vi "n get waveform.vi"(7 "memptr":i16, 8 "error in (no error)":errorcluster, 9 "stopp":u16, 10 "channel":u16, 11 "n":u16) -> (0 "error out":errorcluster, 5 "memptr out":i16)   [LabVIEW 2015, in "SCANalone4x64.lvlib"]
doc: "__declspec(dllimport) void __stdcall n_get_waveform(unsigned short n, unsigned short channel, unsigned short stopp, signed short *memptr);"
uses:
  <userlib>/SCANalone4x64/SCANalone4x64.lvlib
  <userlib>/SCANalone4x64/SCANalone4x64.dll
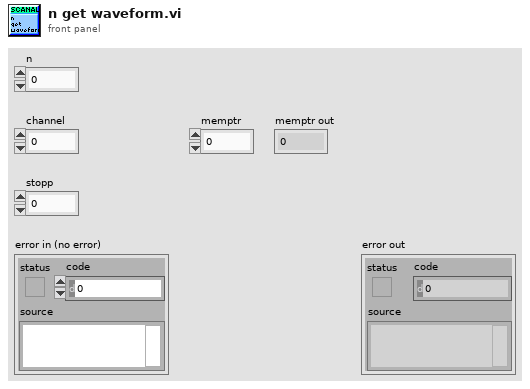
[diagram p1: front panel]
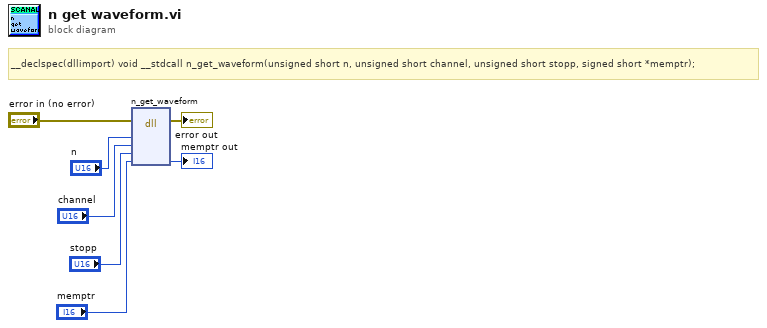
[diagram p0: block diagram]
diagram:
  # "__declspec(dllimport) void __stdcall n_get_waveform(unsigned short n, unsigned short channel, unsigned short stopp, signed short *memptr);"
  n1 = dll-call lib="C:/Program Files/National Instruments/LabVIEW 2015/user.lib/SCANalone4x64/SCANalone4x64.*" fn="n_get_waveform"(error in="error in (no error)", "n"="n", "channel"="channel", "stopp"="stopp", "memptr"="memptr") -> (error out=→"error out":errorcluster, "memptr"=→"memptr out":i16)  [unwired: 6 in, 1 out]
